vi "Drive Base.vi"   [LabVIEW 2018]
uses:
  RefNumsDriverStation.vi
  Motor Power.vi
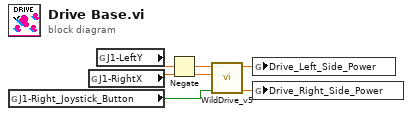
[diagram p0: block diagram]
diagram:
  n1 = global read "RefNumsDriverStation.vi" "J1-Right_Joystick_Button"() -> (w4:bool)
  n2 = global read "RefNumsDriverStation.vi" "J1-RightX"() -> (w5:dbl)
  n3 = global read "RefNumsDriverStation.vi" "J1-LeftY"() -> (w6:dbl)
  n4 = Negate(x=w6) -> (-x=w1:dbl)
  n5 = call "WildDrive_v5.vi"("Super Turn"=w4, "Turn Joystick"=w5, "Speed Joystick"=w1) -> ("Right Side Power"=w2:dbl, "Left Side Power"=w3:dbl)  [unwired: 7 in]
  n6 = global write "Motor Power.vi" "Drive_Left_Side_Power"(w3) -> ()
  n7 = global write "Motor Power.vi" "Drive_Right_Side_Power"(w2) -> ()
